vi "PM100D_Single_Value_ph.vi"(2 "Averaging Period (s)":dbl=1.0, 3 "Beam Name":string="Green Unshifted") -> (0 "Status":T1, 1 "Light Power mW":dbl=8.10606551e-08 format="%^#_9e")   [LabVIEW 2010]
doc: "This VI shows how to communicate with a PM100D optical power/energy meter with SCPI commands.\n- Initializing the instrument\n- Getting system info\n- Setting parameters\n- Measurement configuration\n- Measuring queue\n- Fetching and displaying a measurement value\n- Closing the application"
uses:
  Gen Trav/Multi_Run_Status.ctl
panel:
  out "Wavelength nm":string="488"
  out "IDN String":string="Thorlabs,PM100USB,P2000214,1.3.0\n"
  out "Sensor SN":string="10020635"
  out "Sensor Name":string="S121C"
  out "Sensor Flags":bool[](array[boolean])=[TRUE, FALSE, FALSE, FALSE, FALSE, TRUE, FALSE, FALSE, TRUE, FALSE, FALSE, FALSE, FALSE, FALSE, FALSE, FALSE, FALSE, FALSE, FALSE, FALSE, FALSE, FALSE, FALSE, FALSE, FALSE, FALSE, FALSE, FALSE, FALSE, FALSE, FALSE, FALSE]
  out "New":bool=TRUE
  out "Timeout [ms]":i32=3000
  in  "Readout Config":string(combo)="POW"
  out "Readout string":string="81.06nW"
  out "Error log":string
  out "Averaging Rate":i32=2000
  # "1 Power Sensor"
  # "2 Energy Sensor"
  # "4"
  # "8"
  # "16 Response settable"
  # "32 Wavelength settable"
  # "64 Tau (time constant) settable"
  # "128"
  # "256 With temperature sensor"
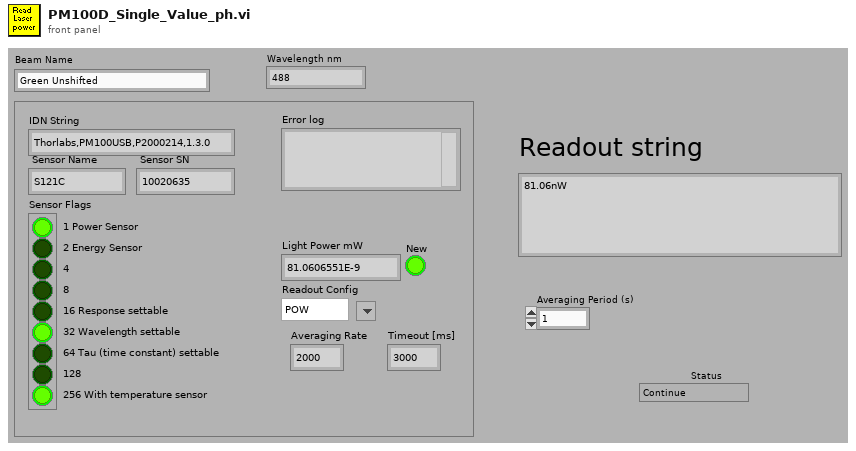
[diagram p1: front panel]
types:
  T1 = typedef "Multi_Run_Status.ctl" = enum16{"Continue", "Jump to Next Point", "Jump to Next Row", "Jump To Fall Back", "Terminate Run"}
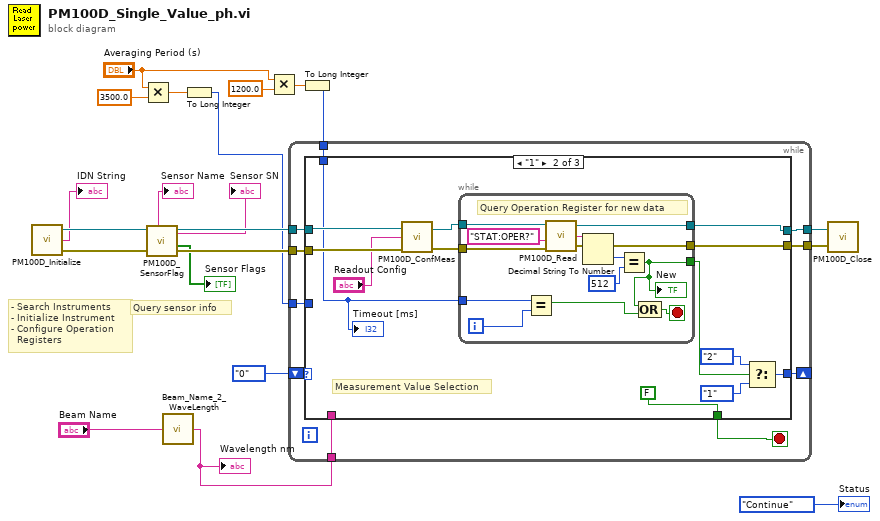
[diagram p0: block diagram]
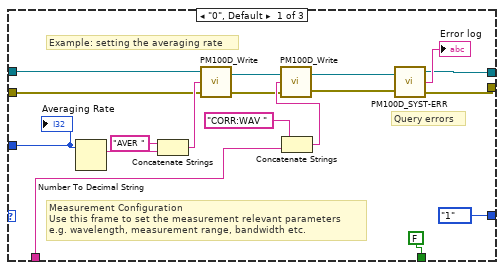
[diagram p2: hidden frame]
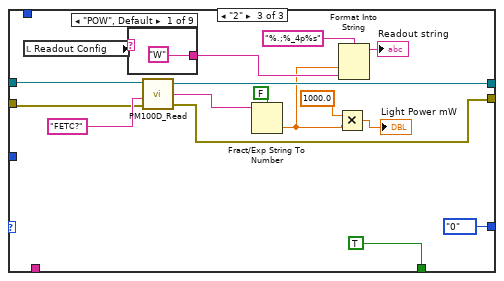
[diagram p3: hidden frame]
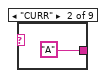
[diagram p4: hidden frame]
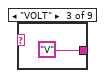
[diagram p5: hidden frame]
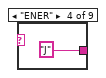
[diagram p6: hidden frame]
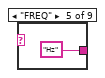
[diagram p7: hidden frame]
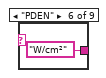
[diagram p8: hidden frame]
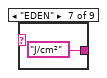
[diagram p9: hidden frame]
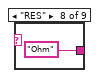
[diagram p10: hidden frame]
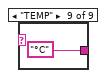
[diagram p11: hidden frame]
diagram:
  # "- Search Instruments\n- Initialize Instrument\n- Configure Operation\n  Registers"
  # "Query sensor info"
  n1 = call "PM100D_Initialize.vi"() -> ("error out"=w20:errorcluster, "Instrument"=→"IDN String":string, "VISA out"=w21:refnum<visa-resource-name>)  [unwired: 3 out]
  n2 = Multiply(x="Averaging Period (s)", y=3500.0) -> (x*y=w6:dbl)
  n3 = call "PM100D_SensorFlag.vi"("error in (no error)"=w20, "VISA in"=w21) -> ("error out"=w18:errorcluster, "flags"=→"Sensor Flags":bool[], "VISA out"=w19:refnum<visa-resource-name>, "sn"=→"Sensor SN":string, "name"=→"Sensor Name":string)  [unwired: 5 out]
  n4 = call "Beam_Name_2_WaveLength.vi"("Beam Name"="Beam Name") -> ("Wavelength nm"=w8:string)
  "Wavelength nm" <- w8
  n5 = To Long Integer(number=w6) -> (32bit integer=w5:i32)
  n6 = Multiply(x="Averaging Period (s)", y=1200.0) -> (x*y=w2:dbl)
  n7 = To Long Integer(number=w2) -> (32bit integer=w1:i32)
  n8 = while {
    tunnel: w19 -> [w31]
    tunnel: w18 -> [w30]
    shift-right: [w28] -> _
    shift-left: enum16{"0", "1", "2"}."0" -> [w29]
    tunnel: [w27] -> w12
    tunnel: [w26] -> w11
    tunnel: w8 -> [w24]
    tunnel: w5 -> [w23]
    tunnel: w1 -> [w22]
    stop <- w25 stop-if-true
    n9 = case shown="\"1\"" w29 {
      tunnel: w31 -> [w47 w62 w89]
      tunnel: w30 -> [w44 w61 w88]
      tunnel: [enum16{"0", "1", "2"}."1" w56 enum16{"0", "1", "2"}."0"] -> w28
      tunnel: [w42 w58 w87] -> w27
      tunnel: [w41 w57 w80] -> w26
      tunnel: [FALSE FALSE TRUE] -> w25
      tunnel: w24 -> [w37 _ _]
      tunnel: w23 -> [w32 _ _]
      tunnel: w22 -> [_ w50 _]
      frame "0", Default {
        # "Query errors"
        # "Example: setting the averaging rate"
        # "Measurement Configuration\nUse this frame to set the measurement relevant parameters\ne.g. wavelength, measurement range, bandwidth etc."
        n10 = Number To Decimal String(number=w32) -> (decimal integer string=w48:string)  [unwired: 1 out]
        n11 = Concatenate Strings("AVER " ("string"), w48) -> (w46:string)
        n12 = call "PM100D_Write.vi"("error in (no error)"=w44, "Command"=w46, "VISA in"=w47) -> ("error out"=w34:errorcluster, "VISA out"=w39:refnum<visa-resource-name>)
        n13 = Concatenate Strings("CORR:WAV " ("string"), w37) -> (w35:string)
        n14 = call "PM100D_Write.vi"("error in (no error)"=w34, "Command"=w35, "VISA in"=w39) -> ("error out"=w33:errorcluster, "VISA out"=w38:refnum<visa-resource-name>)
        n15 = call "PM100D_SYST-ERR.vi"("error out 2"=w33, "VISA In"=w38) -> ("error out"=w41:errorcluster, "Error"=→"Error log":string, "VISA Out"=w42:refnum<visa-resource-name>)  [unwired: 1 out]
        "Averaging Rate" <- w32
      }
      frame "1" {
        # "Measurement Value Selection"
        n16 = call "PM100D_ConfMeas.vi"("error in"=w61, "Conf:"="Readout Config", "VISA In"=w62) -> ("error out"=w59:errorcluster, "dup VISA session"=w60:refnum<visa-resource-name>)
        n17 = while {
          tunnel: w60 -> [w71]
          tunnel: w59 -> [w70]
          tunnel: [w69] -> w58
          tunnel: [w68] -> w57
          tunnel: [w64] -> w53
          tunnel: w50 -> [w63]
          i -> [w66]
          stop <- w67 stop-if-true
          # "Query Operation Register for new data"
          n18 = Equal?(x=w63, y=w66) -> (x = y?=w65:bool)
          n19 = call "PM100D_Read.vi"("error in (no error)"=w70, "Command"="STAT:OPER?", "VISA in"=w71) -> ("error out"=w68:errorcluster, "ReadValue"=w74:string, "VISA out"=w69:refnum<visa-resource-name>)  [unwired: 1 out]
          n20 = Decimal String To Number(string=w74) -> (number=w73:i32)  [unwired: 1 in, 2 out]
          n21 = Equal?(x=w73, y=512) -> (x = y?=w64:bool)
          "New" <- w64
          n22 = Compound Arithmetic op=OR(w64, w65) -> (w67:bool)
        }
        n23 = Select(t=enum16{"0", "1", "2"}."2", s=w53, f=enum16{"0", "1", "2"}."1") -> (s? t:f=w56:enum16{"0", "1", "2"})
        "Timeout [ms]" <- w50
      }
      frame "2" {
        n24 = local read "Readout Config"() -> (w86:string)
        n25 = case shown="\"POW\", Default" w86 {
          tunnel: ["W" "A" "V" "J" "Hz" "W/cm²" "J/cm²" "Ohm" "°C"] -> w82
          frame "POW", Default {
          }
          frame "CURR" {
          }
          frame "VOLT" {
          }
          frame "ENER" {
          }
          frame "FREQ" {
          }
          frame "PDEN" {
          }
          frame "EDEN" {
          }
          frame "RES" {
          }
          frame "TEMP" {
          }
        }
        n26 = call "PM100D_Read.vi"("error in (no error)"=w88, "Command"="FETC?", "VISA in"=w89) -> ("error out"=w80:errorcluster, "ReadValue"=w85:string, "VISA out"=w87:refnum<visa-resource-name>)  [unwired: 1 out]
        n27 = Fract/Exp String To Number(use system decimal point (T)=FALSE, string=w85) -> (number=w77:dbl)  [unwired: 3 out]
        n28 = Multiply(x=1000.0, y=w77) -> (x*y=→"Light Power mW":dbl)
        n29 = Format Into String(format string="%.;%_4p%s", w77, w82) -> (resulting string=→"Readout string":string)  [unwired: 2 in, 1 out]
      }
    }
  }
  n30 = call "PM100D_Close.vi"("error in (no error)"=w11, "VISA resource name"=w12) -> ()  [unwired: 1 in, 1 out]
  "Status" <- Multi_Run_Status."Continue" ("Status")
